vi "FPGA-test001.vi"() -> ()   [LabVIEW 2019]
uses:
  smallmom-3 FPGA test/FPGA-test/Sub VIs/Utilities/Start Boolean.ctl
  <vilib>/Platform/TimedLoop/XDataNode/timing_clust.ctl
  <vilib>/Platform/TimedLoop/XDataNode/nitl_modes.ctl
  <vilib>/Platform/TimedLoop/XDataNode/wakeup.ctl
  <vilib>/rvi/Emulation/niFpgaGetClockAttributes.vi
  <vilib>/rvi/Emulation/niFpgaSctlEmulationGetInTimedLoop.vi
  <vilib>/rvi/Emulation/niFpgaEmulationReportErrorSimple.vi
  <vilib>/rvi/eio/common/nirviEmuTemplateMethod_errors.vi
  <vilib>/rvi/Emulation/niFpgaCriticalErrorInLSC.vi
  <vilib>/eio/EIONode/EIONode.xnode
  <vilib>/platform/TimedLoop/XDataNode/XDataNode.xnode
  <vilib>/Platform/TimedLoop/XDataNode/XDNodeRunTimeDep.lvlib
panel:
  out "us4.distance":i32
  out "us3.distance":i32
  out "us2.distance":i32
  out "us1.distance":i32
  in  "us4.timeout(us)":i32
  in  "us3.timeout(us)":i32
  in  "us2.timeout(us)":i32
  in  "us1.timeout(us)":i32
  in  "Ultrasonic.IO.Enable":u8 format="%.0b"
  in  "I2C.A.GO":T1
  in  "I2C.A.CNFG":u8=1 format="%08b"
  out "I2C.A.STAT":u8 format="%08b"
  in  "I2C.A.CNTL":u8 format="%08b"
  in  "I2C.A.CNTR":u8=213
  in  "I2C.A.ADDR":u8 format="%08b"
  out "I2C.A.DATI":u8
  in  "I2C.A.DATO":u8
  in  "Ultrasonic.IO.Write":u8
  in  "Ultrasonic.io.DIR":u8
  out "Ultrasonic.io.Read":u8
  out "Basic IO Read":u8
  in  "Basic IO DIR":u8
  in  "Basic IO Write":u8
  out "IR 8":u16
  out "IR 7":u16
  out "IR 6":u16
  out "IR 5":u16
  out "IR 4":u16
  out "IR 3":u16
  out "IR 2":u16
  out "IR 1":u16
  in  "Servo3.pulse(0.05us)":u32
  in  "Servo2.pulse(0.05us)":u32
  in  "Servo1.pulse(0.05us)":u32
  in  "Motor3.encoder_Reset":bool
  out "Motor3.encoder":i32
  in  "Motor3.speed":i64
  in  "Motor3.periode":i64
  in  "Motor3.enable_divider":bool
  in  "Motor3.divider":fxp<+,4,4>
  in  "Motor3.brake":bool
  in  "Motor4.encoder_Reset":bool
  out "Motor4.encoder":i32
  in  "Motor4.speed":i64
  in  "Motor4.periode":i64
  in  "Motor4.enable_divider":bool
  in  "Motor4.divider":fxp<+,4,4>
  in  "Motor4.brake":bool
  in  "Motor2.encoder_Reset":bool
  out "Motor2.encoder":i32
  in  "Motor2.speed":i64
  in  "Motor2.periode":i64
  in  "Motor2.enable_divider":bool
  in  "Motor2.divider":fxp<+,4,4>
  in  "Motor2.brake":bool
  in  "Motor1.brake":bool
  in  "Motor1.divider":fxp<+,4,4>
  in  "Motor1.enable_divider":bool
  in  "Motor1.periode":i64
  in  "Motor1.speed":i64
  out "Motor1.encoder":i32
  in  "Motor1.encoder_Reset":bool
  out "OnBoard.BUTTON":bool
  in  "OnBoard.LED[3:0]":fxp<+,4,4> format="%.0b"
  # "Motor1"
  # "Motor2"
  # "Motor3"
  # "Motor4"
  # "Servo"
  # "IR Sensor"
  # "Basic IO"
  # "Ultrasonic IO"
  # "I2C"
  # "OnBoard"
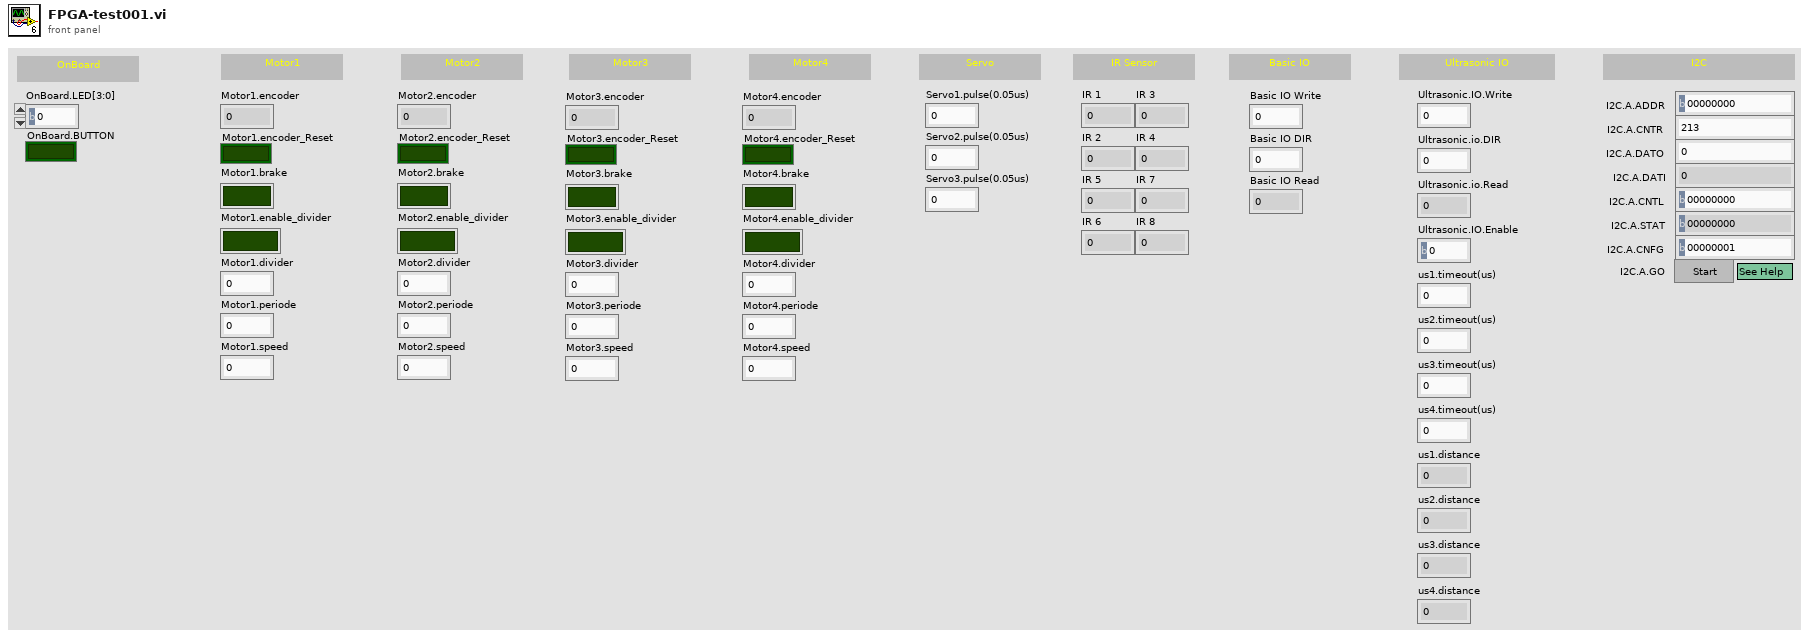
[diagram p1: front panel]
types:
  T1 = typedef "Start Boolean.ctl" = bool
  T2 = typedef "XDNodeRunTimeDep.lvlib/timing_clust.ctl" = cluster{"Expected End [f-1]":u64, "Actual End [f-1]":u64, "Finished Late? [f-1]":bool, "Expected End [i-1]":u64, "Actual End [i-1]":u64, "Finished Late? [i-1]":bool, "Expected Start [i]":u64, "Actual Start [i]":u64, "Expected Start [f]":u64, "Actual Start [f]":u64, "Source Name":string, "Structure Name":string, "Period":i64, "Deadline":i64, "Offset":i64, "Start":i64, "Priority":i32, "Timeout":i32, "Mode":T3, "Wakeup Reason":T4, "Error":errorcluster, "Source Type":string, "Secondary Source Type":string, "Global End Time":u64, "Global Start Time":u64, "Frame Duration":u64, "Iteration Duration":u64, "Assigned CPU":i32, "I/O Scan Engine Mode":u32}
  T3 = typedef "XDNodeRunTimeDep.lvlib/nitl_modes.ctl" = enum32{"No Change", "Process missed periods, maintain original phase", "Discard missed periods, maintain original phase", "Process missed periods, ignore original phase", "Discard missed periods, ignore original phase"}
  T4 = typedef "XDNodeRunTimeDep.lvlib/wakeup.ctl" = enum32{"Normal", "Aborted", "Asynchronous wakeup", "Timing source error", "Timed loop error", "Timeout"}
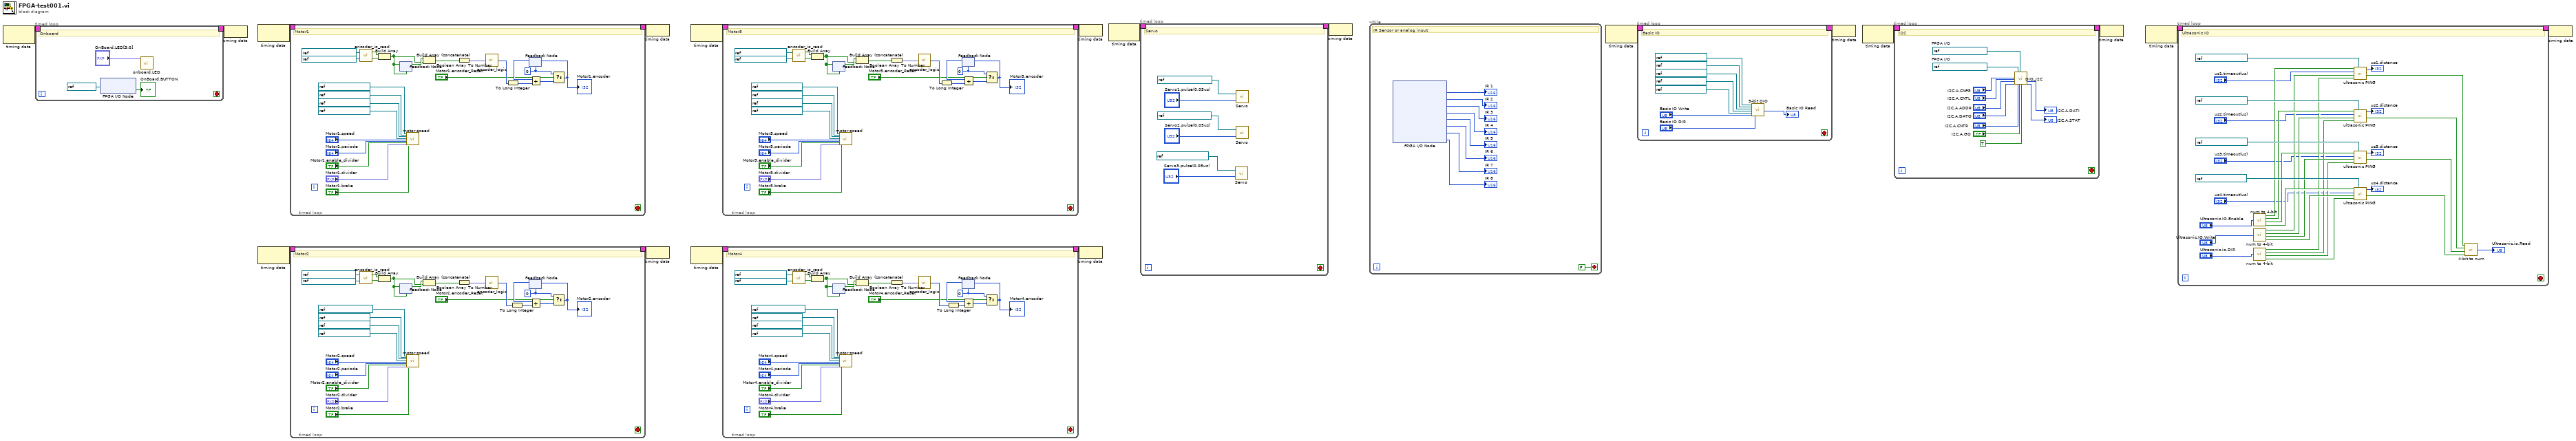
[diagram p0: block diagram]
diagram:
  n1 = node-c288() -> (w18:T2)  [unwired: 1 in]
  n2 = timed-loop "Timed Loop" {
    timing: w18 -> [_]
    timing-out: [_] -> w17
    stop <- _ stop-if-true
    # "Onboard"
    n3 = xnode "FPGA I/O Node"("FPGA I/O In"=refnum<k21> "Button0") -> ("I/O Item"=→"OnBoard.BUTTON":bool)  [unwired: 1 out]
    n4 = call "onboard.LED.vi"("OnBoard.LED[3:0]"="OnBoard.LED[3:0]") -> ()  [unwired: 11 in]
  }
  n5 = node-c288(w17) -> ()
  n6 = node-c288() -> (w16:T2)  [unwired: 1 in]
  n7 = node-c288() -> (w14:T2)  [unwired: 1 in]
  n8 = timed-loop "Timed Loop" {
    timing: w16 -> [_]
    timing-out: [_] -> w15
    stop <- _ stop-if-true
    w38 = 0
    # "Motor1"
    n9 = call "encoder_io_read.vi"("PhaseB"=refnum<k21> "ConnectorA/DIO12", "PhaseA"=refnum<k21> "ConnectorA/DIO11") -> ("PhaseB"=w45:bool, "PhaseA"=w46:bool)
    n10 = Build Array(w46, w45) -> (w43:bool[])
    n11 = feedback-in #1(w43) -> ()
    n12 = feedback #1(w43) -> (w44:bool[])
    n13 = call "motor speed.vi"("IN_A"=refnum<k21> "ConnectorA/DIO2" ("PhaseA"), "IN_B"=refnum<k21> "ConnectorA/DIO0" ("PhaseB"), "Enable"=refnum<k21> "ConnectorA/DIO1" ("PhaseA"), "PWM"=refnum<k21> "ConnectorA/DIO8" ("PhaseB"), "speed"="Motor1.speed", "periode"="Motor1.periode", "enable divider"="Motor1.enable_divider", "divider"="Motor1.divider", "brake"="Motor1.brake") -> ()  [unwired: 19 in]
    n14 = Build Array (concatenate)(w44, w43) -> (w34:bool[])
    n15 = Boolean Array To Number(Boolean array=w34) -> (number=w42:fxp<+,4,4>)
    n16 = call "encoder_logic.vi"("encoder"=w42) -> ("out"=w40:i16)
    n17 = To Long Integer(number=w40) -> (32bit integer=w24:i32)
    n18 = feedback #2(w38) -> (w41:i32)
    n19 = Add(x=w41, y=w24) -> (x+y=w37:i32)
    n20 = Select(t=w38, s="Motor1.encoder_Reset", f=w37) -> (s? t:f=w36:i32)
    "Motor1.encoder" <- w36
    n21 = feedback-in #2(w36) -> ()
  }
  n22 = timed-loop "Timed Loop" {
    timing: w14 -> [_]
    timing-out: [_] -> w13
    stop <- _ stop-if-true
    w64 = 0
    # "Motor2"
    n23 = call "encoder_io_read.vi"("PhaseB"=refnum<k21> "ConnectorB/DIO12", "PhaseA"=refnum<k21> "ConnectorB/DIO11") -> ("PhaseB"=w71:bool, "PhaseA"=w72:bool)
    n24 = Build Array(w72, w71) -> (w69:bool[])
    n25 = feedback-in #3(w69) -> ()
    n26 = feedback #3(w69) -> (w70:bool[])
    n27 = call "motor speed.vi"("IN_A"=refnum<k21> "ConnectorA/DIO13" ("PhaseA"), "IN_B"=refnum<k21> "ConnectorA/DIO3" ("PhaseB"), "Enable"=refnum<k21> "ConnectorA/DIO4" ("PhaseA"), "PWM"=refnum<k21> "ConnectorA/DIO9" ("PhaseB"), "speed"="Motor2.speed", "periode"="Motor2.periode", "enable divider"="Motor2.enable_divider", "divider"="Motor2.divider", "brake"="Motor2.brake") -> ()  [unwired: 19 in]
    n28 = Build Array (concatenate)(w70, w69) -> (w60:bool[])
    n29 = Boolean Array To Number(Boolean array=w60) -> (number=w68:fxp<+,4,4>)
    n30 = call "encoder_logic.vi"("encoder"=w68) -> ("out"=w66:i16)
    n31 = To Long Integer(number=w66) -> (32bit integer=w50:i32)
    n32 = feedback #4(w64) -> (w67:i32)
    n33 = Add(x=w67, y=w50) -> (x+y=w63:i32)
    n34 = Select(t=w64, s="Motor2.encoder_Reset", f=w63) -> (s? t:f=w62:i32)
    "Motor2.encoder" <- w62
    n35 = feedback-in #4(w62) -> ()
  }
  n36 = node-c288(w15) -> ()
  n37 = node-c288(w13) -> ()
  n38 = node-c288() -> (w12:T2)  [unwired: 1 in]
  n39 = node-c288() -> (w10:T2)  [unwired: 1 in]
  n40 = timed-loop "Timed Loop" {
    timing: w12 -> [_]
    timing-out: [_] -> w11
    stop <- _ stop-if-true
    w90 = 0
    # "Motor3"
    n41 = call "encoder_io_read.vi"("PhaseB"=refnum<k21> "ConnectorC/DIO2", "PhaseA"=refnum<k21> "ConnectorC/DIO0") -> ("PhaseB"=w97:bool, "PhaseA"=w98:bool)
    n42 = Build Array(w98, w97) -> (w95:bool[])
    n43 = feedback-in #5(w95) -> ()
    n44 = feedback #5(w95) -> (w96:bool[])
    n45 = call "motor speed.vi"("IN_A"=refnum<k21> "ConnectorB/DIO2" ("PhaseA"), "IN_B"=refnum<k21> "ConnectorB/DIO0" ("PhaseB"), "Enable"=refnum<k21> "ConnectorB/DIO1" ("PhaseA"), "PWM"=refnum<k21> "ConnectorB/DIO8" ("PhaseB"), "speed"="Motor3.speed", "periode"="Motor3.periode", "enable divider"="Motor3.enable_divider", "divider"="Motor3.divider", "brake"="Motor3.brake") -> ()  [unwired: 19 in]
    n46 = Build Array (concatenate)(w96, w95) -> (w86:bool[])
    n47 = Boolean Array To Number(Boolean array=w86) -> (number=w94:fxp<+,4,4>)
    n48 = call "encoder_logic.vi"("encoder"=w94) -> ("out"=w92:i16)
    n49 = To Long Integer(number=w92) -> (32bit integer=w76:i32)
    n50 = feedback #6(w90) -> (w93:i32)
    n51 = Add(x=w93, y=w76) -> (x+y=w89:i32)
    n52 = Select(t=w90, s="Motor3.encoder_Reset", f=w89) -> (s? t:f=w88:i32)
    "Motor3.encoder" <- w88
    n53 = feedback-in #6(w88) -> ()
  }
  n54 = timed-loop "Timed Loop" {
    timing: w10 -> [_]
    timing-out: [_] -> w9
    stop <- _ stop-if-true
    w116 = 0
    # "Motor4"
    n55 = call "encoder_io_read.vi"("PhaseB"=refnum<k21> "ConnectorC/DIO6", "PhaseA"=refnum<k21> "ConnectorC/DIO4") -> ("PhaseB"=w123:bool, "PhaseA"=w124:bool)
    n56 = Build Array(w124, w123) -> (w121:bool[])
    n57 = feedback-in #7(w121) -> ()
    n58 = feedback #7(w121) -> (w122:bool[])
    n59 = call "motor speed.vi"("IN_A"=refnum<k21> "ConnectorB/DIO13" ("PhaseA"), "IN_B"=refnum<k21> "ConnectorB/DIO3" ("PhaseB"), "Enable"=refnum<k21> "ConnectorB/DIO4" ("PhaseA"), "PWM"=refnum<k21> "ConnectorB/DIO9" ("PhaseB"), "speed"="Motor4.speed", "periode"="Motor4.periode", "enable divider"="Motor4.enable_divider", "divider"="Motor4.divider", "brake"="Motor4.brake") -> ()  [unwired: 19 in]
    n60 = Build Array (concatenate)(w122, w121) -> (w112:bool[])
    n61 = Boolean Array To Number(Boolean array=w112) -> (number=w120:fxp<+,4,4>)
    n62 = call "encoder_logic.vi"("encoder"=w120) -> ("out"=w118:i16)
    n63 = To Long Integer(number=w118) -> (32bit integer=w102:i32)
    n64 = feedback #8(w116) -> (w119:i32)
    n65 = Add(x=w119, y=w102) -> (x+y=w115:i32)
    n66 = Select(t=w116, s="Motor4.encoder_Reset", f=w115) -> (s? t:f=w114:i32)
    "Motor4.encoder" <- w114
    n67 = feedback-in #8(w114) -> ()
  }
  n68 = node-c288(w11) -> ()
  n69 = node-c288(w9) -> ()
  n70 = node-c288() -> (w8:T2)  [unwired: 1 in]
  n71 = timed-loop {
    timing: w8 -> [_]
    timing-out: [_] -> w7
    stop <- _ stop-if-true
    # "Servo"
    n72 = call "Servo.vi"("(2.5us)"="Servo3.pulse(0.05us)", "Servo DIO"=refnum<k21> "ConnectorC/DIO3") -> ()  [unwired: 1 in]
    n73 = call "Servo.vi"("(2.5us)"="Servo1.pulse(0.05us)", "Servo DIO"=refnum<k21> "ConnectorA/DIO10") -> ()  [unwired: 1 in]
    n74 = call "Servo.vi"("(2.5us)"="Servo2.pulse(0.05us)", "Servo DIO"=refnum<k21> "ConnectorB/DIO10") -> ()  [unwired: 1 in]
  }
  n75 = node-c288(w7) -> ()
  n76 = while {
    stop <- FALSE stop-if-true
    # "IR Sensor or analog input"
    n77 = xnode "FPGA I/O Node"() -> ("ConnectorA/AI3"=→"IR 1":u16, "ConnectorA/AI2"=→"IR 2":u16, "ConnectorA/AI1"=→"IR 3":u16, "ConnectorA/AI0"=→"IR 4":u16, "ConnectorB/AI3"=→"IR 5":u16, "ConnectorB/AI2"=→"IR 6":u16, "ConnectorB/AI1"=→"IR 7":u16, "ConnectorB/AI0"=→"IR 8":u16)  [unwired: 8 in, 8 out]
  }
  n78 = node-c288() -> (w6:T2)  [unwired: 1 in]
  n79 = timed-loop {
    timing: w6 -> [_]
    timing-out: [_] -> w5
    stop <- _ stop-if-true
    # "Basic IO"
    n80 = call "5-bit DIO.vi"("DIO Refnum 1"=refnum<k21> "ConnectorC/DIO1", "DIO Refnum 2"=refnum<k21> "ConnectorC/DIO5" ("DIO Refnum 1"), "DIO Refnum 3"=refnum<k21> "ConnectorC/DIO7" ("DIO Refnum 1"), "DIO Refnum 4"=refnum<k21> "ConnectorB/DIO6" ("DIO Refnum 1"), "DIO Refnum 5"=refnum<k21> "ConnectorB/DIO7" ("DIO Refnum 1"), "DIO OUT[4:0]"="Basic IO Write", "DIO DIR[4:0]"="Basic IO DIR") -> ("DIO IN[4:0]"=→"Basic IO Read":u8)  [unwired: 12 in]
  }
  n81 = node-c288(w5) -> ()
  n82 = node-c288() -> (w2:T2)  [unwired: 1 in]
  n83 = timed-loop {
    timing: w2 -> [_]
    timing-out: [_] -> w1
    stop <- _ stop-if-true
    w156 = refnum<k21> "ConnectorA/DIO15"  # FPGA I/O
    w157 = refnum<k21> "ConnectorA/DIO14"  # FPGA I/O
    # "I2C"
    n84 = call "DIO_I2C.vi"("I2C.CNFG"="I2C.A.CNFG", "I2C.CNTL"="I2C.A.CNTL", "I2C.ADDR"="I2C.A.ADDR", "I2C.DATO"="I2C.A.DATO", "DIO.1/I2C.SDA"=w156, "I2C.CNTR"="I2C.A.CNTR", "DIO.0/I2C.SCL"=w157, "Execute?"="I2C.A.GO", "SELECT"=TRUE) -> ("I2C.DATI"=→"I2C.A.DATI":u8, "I2C.STAT"=→"I2C.A.STAT":u8)  [unwired: 8 in, 1 out]
  }
  n85 = node-c288(w1) -> ()
  n86 = node-c288() -> (w4:T2)  [unwired: 1 in]
  n87 = timed-loop {
    timing: w4 -> [_]
    timing-out: [_] -> w3
    stop <- _ stop-if-true
    # "Ultrasonic IO"
    n88 = call "num to 4-bit.vi"("DIO DIR[3:0]"="Ultrasonic.IO.Enable") -> ("element"=w192:bool, "element 2"=w191:bool, "element 3"=w190:bool, "element 4"=w189:bool)
    n89 = call "num to 4-bit.vi"("DIO DIR[3:0]"="Ultrasonic.IO.Write") -> ("element"=w188:bool, "element 2"=w187:bool, "element 3"=w186:bool, "element 4"=w185:bool)
    n90 = call "num to 4-bit.vi"("DIO DIR[3:0]"="Ultrasonic.io.DIR") -> ("element"=w184:bool, "element 2"=w183:bool, "element 3"=w182:bool, "element 4"=w181:bool)
    n91 = call "ultrasonic PING.vi"("DIO Refnum"=refnum<k21> "ConnectorA/DIO7" ("DIO Refnum 1"), "DIR"=w184, "OUT"=w188, "timeout(us)"="us1.timeout(us)", "F selection"=w192) -> ("IN"=w179:bool, "ultrasonic output"=→"us1.distance":i32)  [unwired: 5 in]
    n92 = call "ultrasonic PING.vi"("DIO Refnum"=refnum<k21> "ConnectorA/DIO6" ("DIO Refnum 1"), "DIR"=w183, "OUT"=w187, "timeout(us)"="us2.timeout(us)", "F selection"=w191) -> ("IN"=w178:bool, "ultrasonic output"=→"us2.distance":i32)  [unwired: 5 in]
    n93 = call "ultrasonic PING.vi"("DIO Refnum"=refnum<k21> "ConnectorA/DIO5" ("DIO Refnum 1"), "DIR"=w182, "OUT"=w186, "timeout(us)"="us3.timeout(us)", "F selection"=w190) -> ("IN"=w177:bool, "ultrasonic output"=→"us3.distance":i32)  [unwired: 5 in]
    n94 = call "ultrasonic PING.vi"("DIO Refnum"=refnum<k21> "ConnectorB/DIO5" ("DIO Refnum 1"), "DIR"=w181, "OUT"=w185, "timeout(us)"="us4.timeout(us)", "F selection"=w189) -> ("IN"=w176:bool, "ultrasonic output"=→"us4.distance":i32)  [unwired: 5 in]
    n95 = call "4-bit to num.vi"("Boolean 4"=w176, "Boolean 3"=w177, "Boolean 2"=w178, "Boolean"=w179) -> ("DIO IN[3:0]"=→"Ultrasonic.io.Read":u8)
  }
  n96 = node-c288(w3) -> ()
